vi "potmeter_voltage_to_erpm.vi"(11 "potmeter_voltage":dbl) -> (2 "greater_than_10?":bool, 3 "e_rpm":dbl)   [LabVIEW 2014]
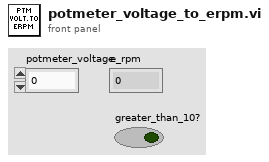
[diagram p1: front panel]
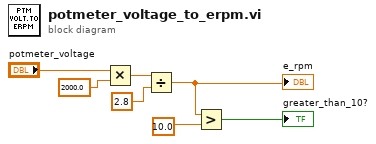
[diagram p0: block diagram]
diagram:
  n1 = Multiply(x="potmeter_voltage", y=2000.0) -> (x*y=w6:dbl)
  n2 = Divide(x=w6, y=2.8) -> (x/y=w1:dbl)
  "e_rpm" <- w1
  n3 = Greater?(x=w1, y=10.0) -> (0:→"greater_than_10?":bool)
